vi "Agilent34420A-V1yV2_v7.0.vi"() -> ()   [LabVIEW 2014]
uses:
  <vilib>/Utility/file.llb/Write To Spreadsheet File (string).vi
  Program Files/National Instruments/LabVIEW 2014/instr.lib/Agilent 34401/Agilent 34401.lvlib
panel:
  out "Medicion CH1":string[](array[string])
  out "Tmed":string[](array[string])
  out "new file path (Not A Path if cancelled)":path
  out "tiempo transcurrido (s)":dbl
  out "tiempo inicio":timestamp format="%<%H:%M:%S%1u>T"
  in  "t esp medic CH1":dbl
  in  "NPLC CH1":sgl(ring)=2.0 format="%_1f" items=["200", "100", "20", "10", "2", "1", ".2", "0.02"]
  in  "RESOL CH1":dbl
  in  "RANGE CH1 (V)":dbl=0.1
  in  "file path (dialog if empty)":path=path "C:/Users/INTI/Desktop/Gonzalo/INTI/Gonzalo/agilent34420_medicion_de_cosa_turbia/mediciones"
  out "Waveform Graph":dbl[](graph)
  out "medic ch 1":dbl[](array[numeric]) format="%#.10e"
  in  "termina medic":bool
  out "Boolean":bool
  in  "empieza medic":bool
  in  "error":errorcluster
  in  "GPIB mult":refnum<visa-resource-name>="GPIB0::13::INSTR"
  # "Notas: el programa mide en forma alternada el canal 1 y 2 del multímetro con los rangos y NPLC seleccionados.\n1- seleccionar GPIB addrs\n2- selccionar RANGE y NPLC de los canales, puede elegirse un file path o dejarlo en blanco (al final se pedirá archivo de datos a grabar).\n3- click en MEDIR para comenzar la medición\n4- click en TERMINAR para finalizarla, se solicita file path en este punto de no haberlo seleccionado previamente."
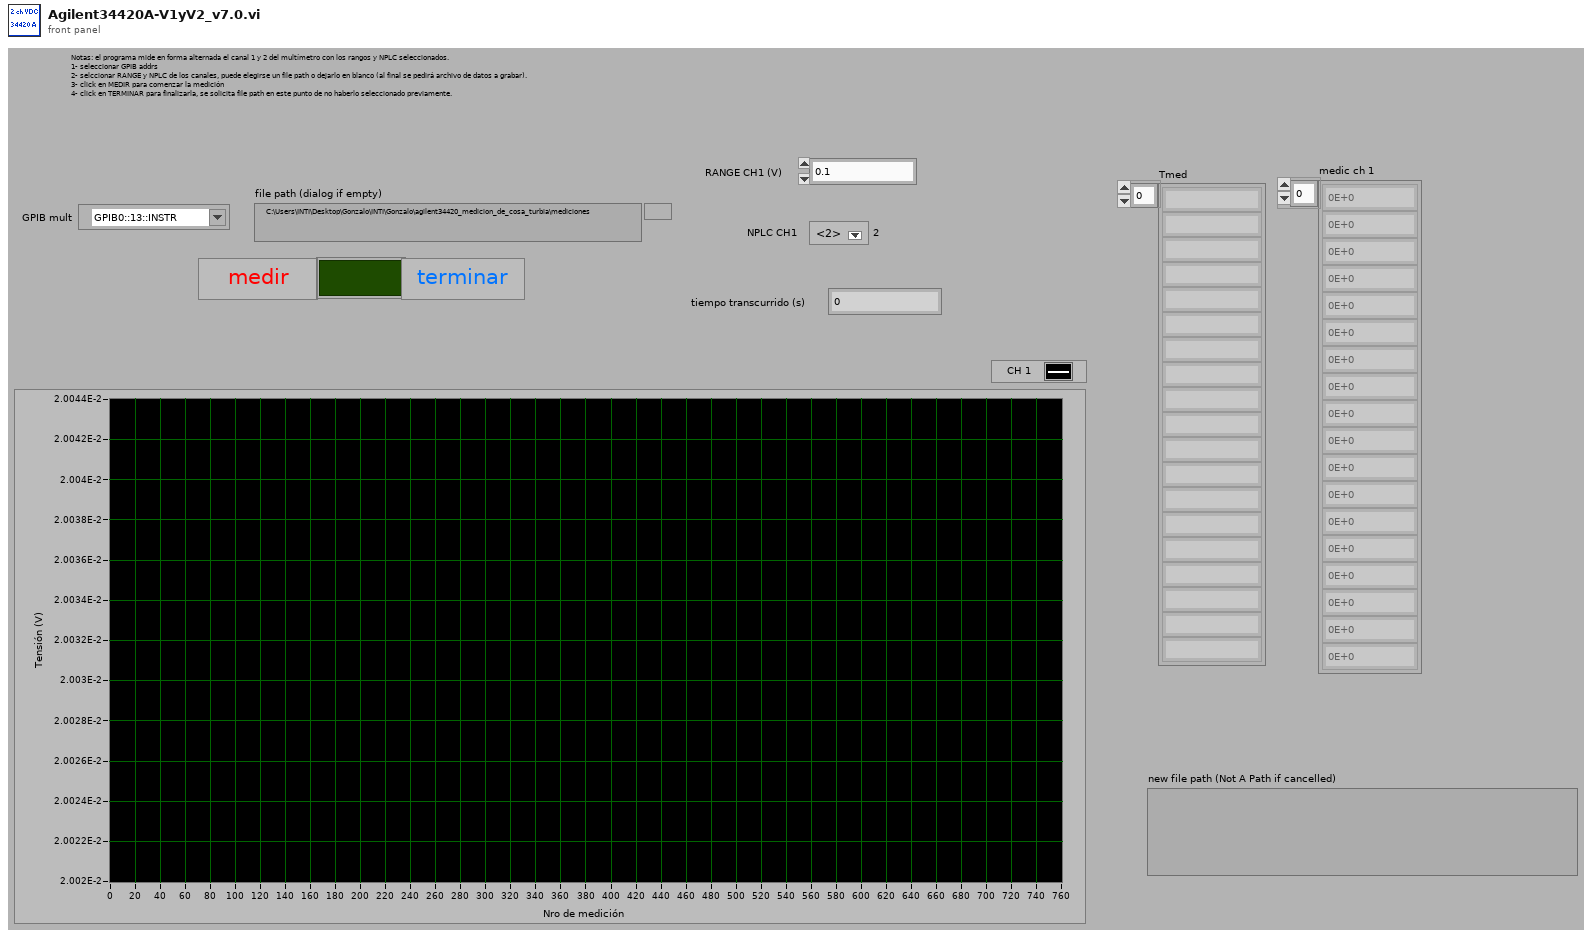
[diagram p1: front panel]
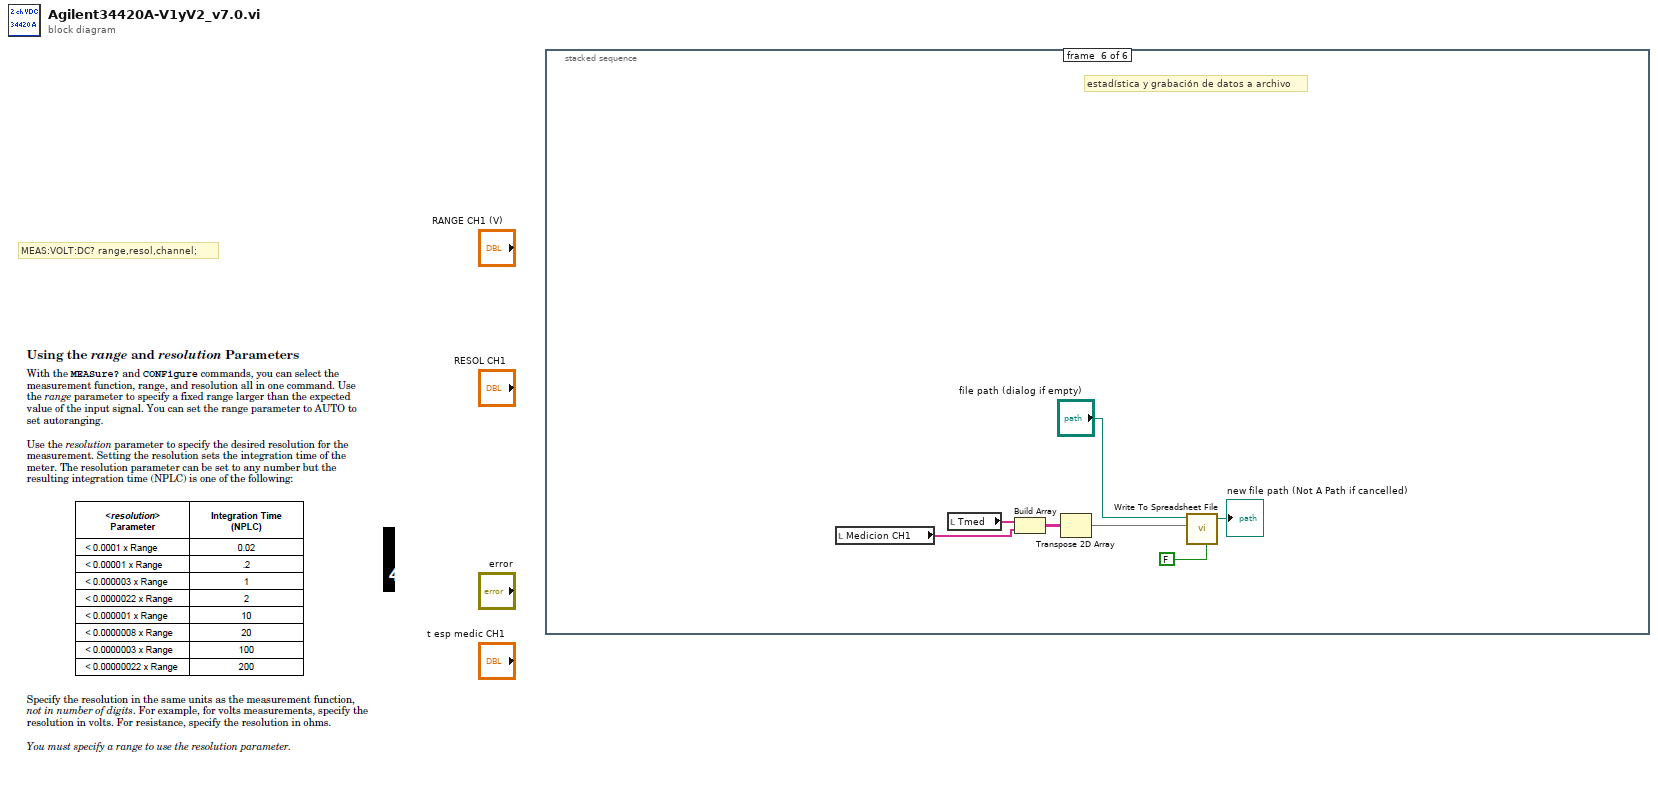
[diagram p0: block diagram]
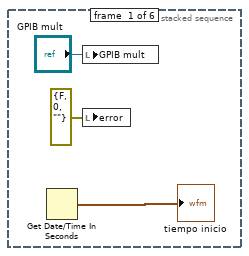
[diagram p2: hidden frame]
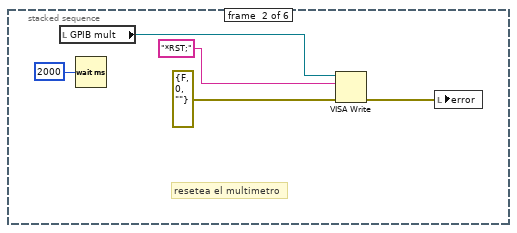
[diagram p3: hidden frame]
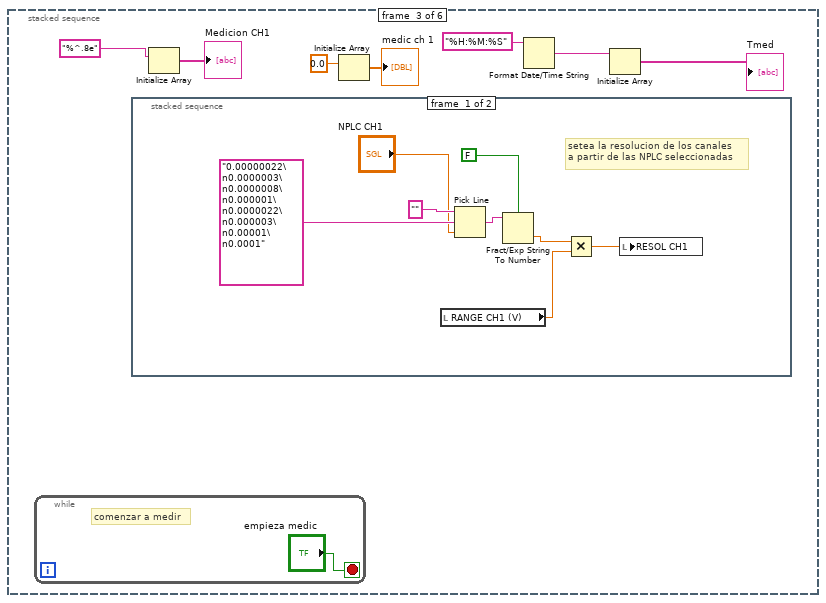
[diagram p4: hidden frame]
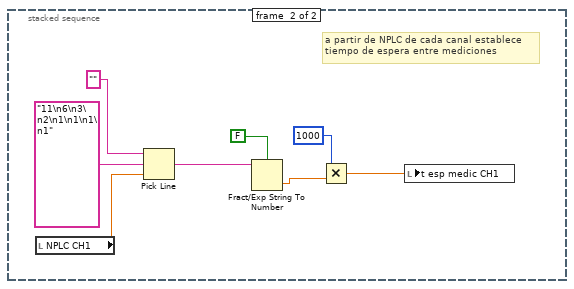
[diagram p5: hidden frame]
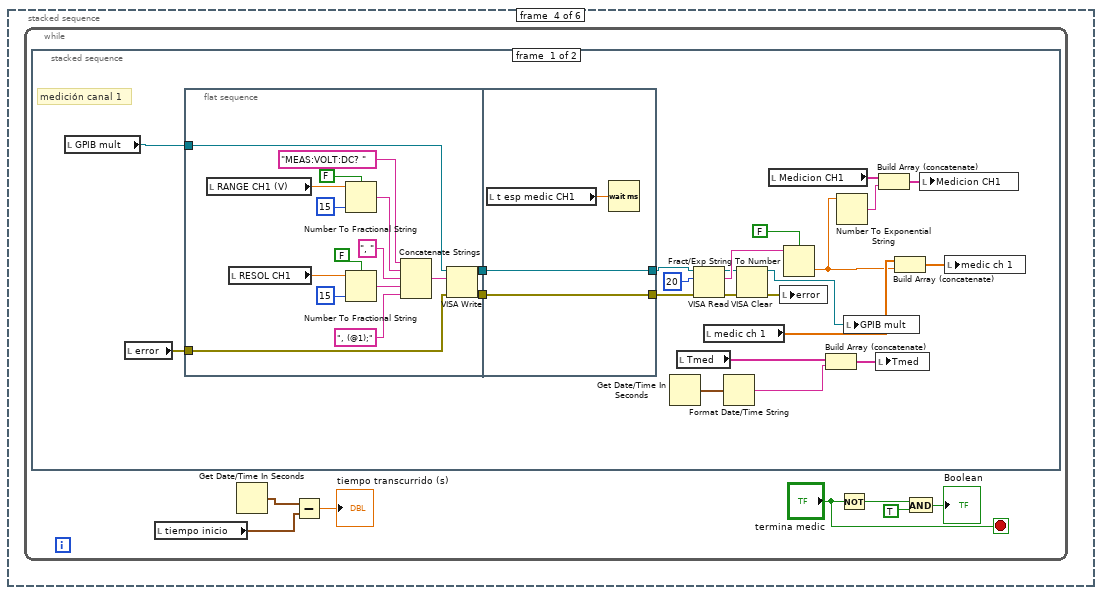
[diagram p6: hidden frame]
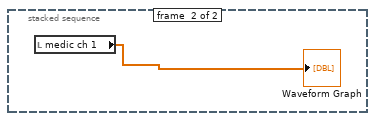
[diagram p7: hidden frame]
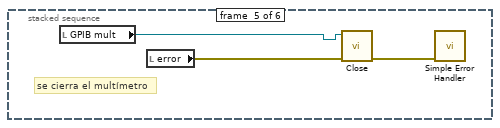
[diagram p8: hidden frame]
diagram:
  # "MEAS:VOLT:DC? range,resol,channel;"
  n1 = stacked-sequence {
    frame #0 {
      n2 = Get Date/Time In Seconds() -> (seconds since 1Jan1904=→"tiempo inicio":timestamp)
      n3 = local write "GPIB mult"("GPIB mult") -> ()
      n4 = local write "error"(errorcluster {"status"=FALSE, "code"=0, "source"=""} ("error in (no error)")) -> ()
    }
    frame #1 {
      # "resetea el multimetro"
      n5 = local read "GPIB mult"() -> (w8:refnum<visa-resource-name>)
      n6 = Wait (ms)(milliseconds to wait=u32 2000) -> ()  [unwired: 1 out]
      n7 = VISA Write(VISA resource name=w8, write buffer="*RST;", error in (no error)=errorcluster {"status"=FALSE, "code"=0, "source"=""}) -> (error out=w5:errorcluster)  [unwired: 2 out]
      n8 = local write "error"(w5) -> ()
    }
    frame #2 {
      n9 = while {
        stop <- "empieza medic" stop-if-true
        # "comenzar a medir"
      }
      n10 = stacked-sequence {
        frame #0 {
          # "setea la resolucion de los canales \na partir de las NPLC seleccionadas"
          n11 = local read "RANGE CH1 (V)"() -> (w23:dbl)
          n12 = Pick Line(string ("")="", multi-line string="0.00000022\n0.0000003\n0.0000008\n0.000001\n0.0000022\n0.000003\n0.00001\n0.0001", line index="NPLC CH1") -> (output string=w18:string)
          n13 = Fract/Exp String To Number(use system decimal point (T)=FALSE, string=w18) -> (number=w17:dbl)  [unwired: 2 in, 1 out]
          n14 = Multiply(x=w17, y=w23) -> (x*y=w22:dbl)
          n15 = local write "RESOL CH1"(w22) -> ()
        }
        frame #1 {
          # "a partir de NPLC de cada canal establece\ntiempo de espera entre mediciones"
          n16 = local read "NPLC CH1"() -> (w24:sgl)
          n17 = Pick Line(string ("")="", multi-line string="11\n6\n3\n2\n1\n1\n1\n1", line index=w24) -> (output string=w31:string)
          n18 = Fract/Exp String To Number(use system decimal point (T)=FALSE, string=w31) -> (number=w28:dbl)  [unwired: 2 in, 1 out]
          n19 = Multiply(x=1000, y=w28) -> (x*y=w26:dbl)
          n20 = local write "t esp medic CH1"(w26) -> ()
        }
      }
      n21 = Initialize Array("%^.8e" ("format (%.3f)")) -> (→"Medicion CH1":string[])  [unwired: 1 in]
      n22 = Initialize Array(0.0 ("element")) -> (→"medic ch 1":dbl[])  [unwired: 1 in]
      n23 = Format Date/Time String(time format string (%c)="%H:%M:%S") -> (date/time string=w13:string)  [unwired: 2 in]
      n24 = Initialize Array(w13) -> (→"Tmed":string[])  [unwired: 1 in]
    }
    frame #3 {
      n25 = while {
        stop <- "termina medic" stop-if-true
        n26 = stacked-sequence {
          frame #0 {
            # "medición canal 1"
            n27 = local read "GPIB mult"() -> (w53:refnum<visa-resource-name>)
            n28 = local read "error"() -> (w54:errorcluster)
            n29 = flat-sequence {
              tunnel: w54 -> [w78]
              tunnel: w53 -> [w77]
              tunnel: [w76] -> w50
              tunnel: [w75] -> w49
              tunnel: [w80] -> w51
              tunnel: [w81] -> w52
              tunnel: w50 -> [w81]
              tunnel: w49 -> [w80]
              frame #0 {
                n30 = local read "RANGE CH1 (V)"() -> (w73:dbl)
                n31 = local read "RESOL CH1"() -> (w68:dbl)
                n32 = Number To Fractional String(use system decimal point (T)=FALSE, number=w73, precision (6)=i16 15) -> (F-format string=w71:string)  [unwired: 1 in]
                n33 = Number To Fractional String(use system decimal point (T)=FALSE, number=w68, precision (6)=i16 15) -> (F-format string=w67:string)  [unwired: 1 in]
                n34 = Concatenate Strings("MEAS:VOLT:DC? " ("write buffer"), w71, ", " ("string"), w67, ", (@1);" ("string")) -> (w65:string)
                n35 = VISA Write(VISA resource name=w77, write buffer=w65, error in (no error)=w78) -> (VISA resource name out=w76:refnum<visa-resource-name>, error out=w75:errorcluster)  [unwired: 1 out]
              }
              frame #1 {
                n36 = local read "t esp medic CH1"() -> (w79:dbl)
                n37 = Wait (ms)(milliseconds to wait=w79) -> ()  [unwired: 1 out]
              }
            }
            n38 = Get Date/Time In Seconds() -> (seconds since 1Jan1904=w44:timestamp)
            n39 = local read "Tmed"() -> (w46:string[])
            n40 = VISA Read(VISA resource name=w52, byte count=u32 20, error in (no error)=w51) -> (VISA resource name out=w60:refnum<visa-resource-name>, read buffer=w62:string, error out=w59:errorcluster)  [unwired: 1 out]
            n41 = local read "medic ch 1"() -> (w61:dbl[])
            n42 = Format Date/Time String(seconds (now)=w44) -> (date/time string=w45:string)  [unwired: 2 in]
            n43 = VISA Clear(VISA resource name=w60, error in (no error)=w59) -> (VISA resource name out=w57:refnum<visa-resource-name>, error out=w58:errorcluster)
            n44 = local read "Medicion CH1"() -> (w42:string[])
            n45 = local write "error"(w58) -> ()
            n46 = Fract/Exp String To Number(use system decimal point (T)=FALSE, string=w62) -> (number=w43:dbl)  [unwired: 2 in, 1 out]
            n47 = Build Array (concatenate)(w46, w45) -> (w47:string[])
            n48 = Number To Exponential String(number=w43) -> (E-format string=w41:string)  [unwired: 3 in]
            n49 = local write "GPIB mult"(w57) -> ()
            n50 = local write "Tmed"(w47) -> ()
            n51 = Build Array (concatenate)(w42, w41) -> (w40:string[])
            n52 = Build Array (concatenate)(w61, w43) -> (w48:dbl[])
            n53 = local write "Medicion CH1"(w40) -> ()
            n54 = local write "medic ch 1"(w48) -> ()
          }
          frame #1 {
            n55 = local read "medic ch 1"() -> (→"Waveform Graph":dbl[])
          }
        }
        n56 = local read "tiempo inicio"() -> (w34:timestamp)
        n57 = Get Date/Time In Seconds() -> (seconds since 1Jan1904=w35:timestamp)
        n58 = Subtract(x=w35, y=w34) -> (x-y=→"tiempo transcurrido (s)":dbl)
        n59 = Not(x="termina medic") -> (.not. x?=w37:bool)
        n60 = And(x=w37, y=TRUE ("Boolean")) -> (x .and. y?=→"Boolean":bool)
      }
    }
    frame #4 {
      # "se cierra el multímetro"
      n61 = local read "GPIB mult"() -> (w85:refnum<visa-resource-name>)
      n62 = local read "error"() -> (w84:errorcluster)
      n63 = call "Close.vi"("error in (no error)"=w84, "VISA resource name"=w85) -> ("error out"=w83:errorcluster)  [unwired: 9 in]
      n64 = call <vilib>:"Simple Error Handler.vi"("error in (no error)"=w83) -> ()  [unwired: 4 in, 5 out]
    }
    frame #5 {
      # "estadística y grabación de datos a archivo"
      n65 = local read "Medicion CH1"() -> (w88:string[])
      n66 = local read "Tmed"() -> (w89:string[])
      n67 = Build Array(w89, w88) -> (w87:string[][])
      n68 = Transpose 2D Array(2D array=w87) -> (transposed array=w86:string[][])
      n69 = call-poly <vilib>:"Write To Spreadsheet File.vi"("transpose? (no:F)"=FALSE, "2D data"=w86, "file path (dialog if empty)"="file path (dialog if empty)") -> ("new file path (Not A Path if cancelled)"=→"new file path (Not A Path if cancelled)":path)  [unwired: 5 in]
    }
  }
